vi "MDPtr Example.vi"() -> ()   [LabVIEW 2014]
uses:
  MDPtr TypeDef/MDPtr SupportedDataTypeDef.ctl
  _PolymorphicVIs/MDPtr Pack DoubleArr.vi
  _PolymorphicVIs/MDPtr Unpack DoubleArr.vi
panel:
  out "Copy Count":i32
  out "Data Type":T1
  out "Value out":i32
  out "error out":errorcluster
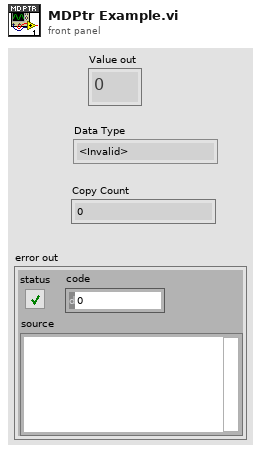
[diagram p1: front panel]
types:
  T1 = typedef "MDPtr SupportedDataTypeDef.ctl" = enum16{"<Invalid>", "Waveform", "Waveform Arr", "Double Arr"}
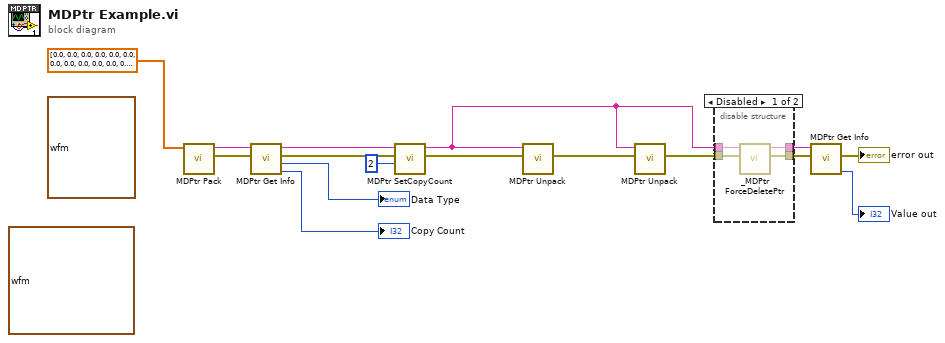
[diagram p0: block diagram]
diagram:
  (unwired) waveform(dbl) {"t0"=timestamp(0 s since 1904-01-01), "dt"=1.0, "Y"=[]} ("waveform")
  (unwired) waveform(dbl)[] [{"t0"=timestamp(0 s since 1904-01-01), "dt"=1.0, "Y"=[]}, {"t0"=timestamp(0 s since 1904-01-01), "dt"=2.0, "Y"=[]}] ("waveforms")
  n1 = call-poly "MDPtr Pack.vi"("Double Array"=dbl[] [0.0, 0.0, 0.0, 0.0, 0.0, 0.0, 0.0, 0.0, 0.0, 0.0, 0.0, 0.0, 0.0, 0.0, 0.0, 0.0, 0.0, 0.0, 0.0, 0.0, 0.0, 0.0, 0.0, 0.0, 0.0, 0.0, 0.0, 0.0, 0.0, 0.0, 0.0, 0.0, 0.0, 0.0, 0.0, 0.0, 0.0, 0.0, 0.0, 0.0, 0.0, 0.0, 0.0, 0.0, 0.0, 0.0, 0.0, 0.0, 0.0, 0.0, 0.0, 0.0, 0.0, 0.0, 0.0, 0.0, 0.0, 0.0, 0.0, 0.0, 0.0, 0.0, 0.0, 0.0, 0.0, 0.0, 0.0, 0.0, 0.0, 0.0, 0.0, 0.0, 0.0, 0.0, 0.0, 0.0, 0.0, 0.0, 0.0, 0.0, 0.0, 0.0, 0.0, 0.0, 0.0, 0.0, 0.0, 0.0, 0.0, 0.0, 0.0, 0.0, 0.0, 0.0, 0.0, 0.0, 0.0, 0.0, 0.0, 0.0, 0.0, 0.0, 0.0, 0.0, 0.0, 0.0, 0.0, 0.0, 0.0, 0.0, 0.0, 0.0, 0.0, 0.0, 0.0, 0.0, 0.0, 0.0, 0.0, 0.0, 0.0, 0.0, 0.0, 0.0, 0.0, 0.0, 0.0, 0.0, 0.0, 0.0, 0.0, 0.0, 0.0, 0.0, 0.0, 0.0, 0.0, 0.0, 0.0, 0.0, 0.0, 0.0, 0.0, 0.0, 0.0, 0.0, 0.0, 0.0, 0.0, 0.0, 0.0, 0.0, 0.0, 0.0, 0.0, 0.0, 0.0, 0.0, 0.0, 0.0, 0.0, 0.0, 0.0, 0.0, 0.0, 0.0, 0.0, 0.0, 0.0, 0.0, 0.0, 0.0, 0.0, 0.0, 0.0, 0.0, 0.0, 0.0, 0.0, 0.0, 0.0, 0.0, 0.0, 0.0, 0.0, 0.0, 0.0, 0.0, 0.0, 0.0, 0.0, 0.0, 0.0, 0.0, 0.0, 0.0, 0.0, 0.0, 0.0, 0.0, 1.0] ("Y")) -> ("error out"=w14:errorcluster, "HexStrPtr"=w15:string)  [unwired: 9 in]
  n2 = call "MDPtr Get Info.vi"("error in (no error)"=w14, "HexStrPtr"=w15) -> ("Copy Count"=→"Copy Count":i32, "Data Type"=→"Data Type":T1, "error out"=w10:errorcluster, "HexStrPtr (dup)"=w11:string)  [unwired: 5 in]
  n3 = call "MDPtr SetCopyCount.vi"("Copy Count"=2, "error in (no error)"=w10, "HexStrPtr"=w11) -> ("error out"=w9:errorcluster, "HexStrPtr (dup)"=w3:string)  [unwired: 6 in]
  n4 = call-poly "MDPtr Unpack.vi"("error in (no error)"=w9, "HexStrPtr"=w3) -> ("error out"=w16:errorcluster)  [unwired: 8 in, 1 out]
  n5 = call-poly "MDPtr Unpack.vi"("error in (no error)"=w16, "HexStrPtr"=w3) -> ("error out"=w7:errorcluster)  [unwired: 8 in, 1 out]
  n6 = disable-structure shown="Disabled" {
    disable-tunnel: w7 -> [w20 w21]
    disable-tunnel: [w19 w21] -> w4
    disable-tunnel: w3 -> [w18 w22]
    disable-tunnel: [w17 w22] -> w2
    frame Disabled {
      n7 = call "_MDPtr ForceDeletePtr.vi"("error in (no error)"=w20, "HexStrPtr"=w18) -> ("error out"=w19:errorcluster, "HexStrPtr (dup)"=w17:string)  [unwired: 7 in]
    }
    frame Enabled {
    }
  }
  n8 = call "MDPtr Get Info.vi"("error in (no error)"=w4, "HexStrPtr"=w2) -> ("Copy Count"=→"Value out":i32, "error out"=→"error out":errorcluster)  [unwired: 5 in, 2 out]
